vi "gTemperature.vi"() -> ()   [LabVIEW 2019]
panel:
  in  "Time-out (s)":dbl=60.0 format="%.3f"
  in  "TempControl Tolerance":dbl=0.1 format="%.3f"
  in  "Manual Advancing?":bool
  in  "Temperature OK?":bool
  in  "Temp (K)":dbl format="%.2f"
  # "Temperature Global Controls"
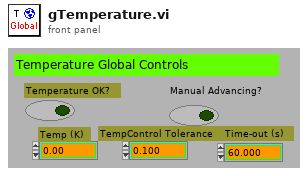
[diagram p1: front panel]
diagram:
